vi "Calculating Acceleration.vi"() -> ()   [LabVIEW 2020]
panel:
  in  "stop":bool
  out "Acceleration (m/s^2)":dbl(knob) scale=0.0..10.0
  in  "Force (N)":dbl(slide) scale=0.0..10.0
  in  "Mass (Kg)":dbl
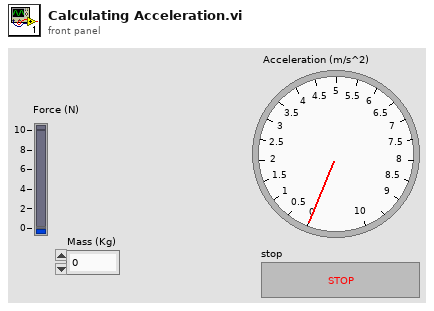
[diagram p1: front panel]
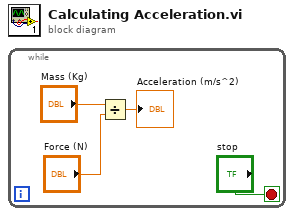
[diagram p0: block diagram]
diagram:
  n1 = while {
    stop <- "stop" stop-if-true
    n2 = Divide(x="Mass (Kg)", y="Force (N)") -> (x/y=→"Acceleration (m/s^2)":dbl)
  }
